vi "Sting to fractional.vi"(11 "String":string) -> (3 "Numeric":dbl)   [LabVIEW 2020]
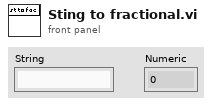
[diagram p1: front panel]
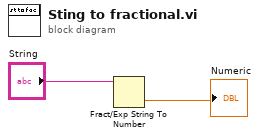
[diagram p0: block diagram]
diagram:
  n1 = Fract/Exp String To Number(string="String") -> (number=→"Numeric":dbl)  [unwired: 3 in, 1 out]
